vi "Configure Timed Output.vi"(8 "error in (no error)":errorcluster, 9 "Time (1s)":dbl=1.0 min=0.0 max=99999.9 step=1.0 format="%.1f", 10 "Enable Timer Output (F: False)":bool, 11 "VISA resource name":refnum<visa-resource-name>) -> (0 "error out":errorcluster, 3 "VISA resource name out":refnum<visa-resource-name>)   [LabVIEW 2016, in "BK Precision 9200 Series.lvlib"]
doc: "Configures and enables the internal output timer."
uses:
  <instrlib>/BK Precision 9200 Series/BK Precision 9200 Series.lvlib
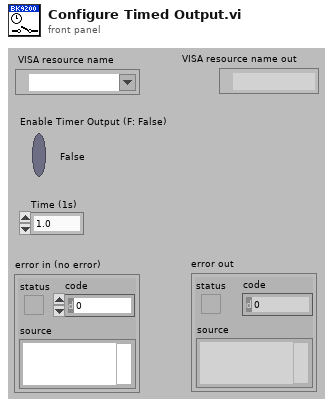
[diagram p1: front panel]
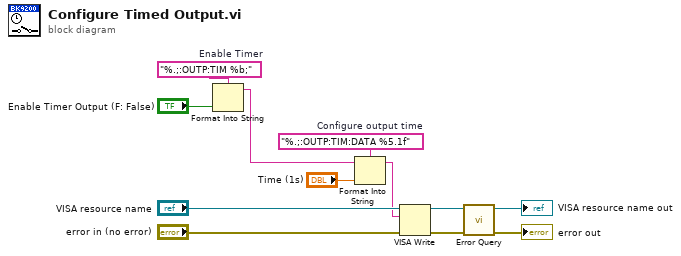
[diagram p0: block diagram]
diagram:
  w5 = "%.;:OUTP:TIM:DATA %5.1f"  # Configure output time
  w10 = "%.;:OUTP:TIM %b;"  # Enable Timer
  n1 = Format Into String(format string=w10, "Enable Timer Output (F: False)") -> (resulting string=w3:string)  [unwired: 2 in, 1 out]
  n2 = Format Into String(format string=w5, initial string=w3, "Time (1s)") -> (resulting string=w2:string)  [unwired: 1 in, 1 out]
  n3 = VISA Write(VISA resource name="VISA resource name", write buffer=w2, error in (no error)="error in (no error)") -> (VISA resource name out=w9:refnum<visa-resource-name>, error out=w8:errorcluster)  [unwired: 1 out]
  n4 = call <instrlib>:"Error Query.vi"("error in (no error)"=w8, "VISA resource name"=w9) -> ("error out"=→"error out":errorcluster, "VISA resource name out"=→"VISA resource name out":refnum<visa-resource-name>)  [unwired: 6 in, 2 out]
